vi "Export - Tx Packets.vi"(8 "error in (no error)":errorcluster, 11 "Device Item Ref in":T5 format="%.0x") -> (0 "error out":errorcluster, 3 "Tx Packets":T1 {"Tx Packet Data"."Endianness" items=["big-endian"=0, "little-endian"=2]})   [LabVIEW 2016, in "UDP-Custom-Device System Explorer.lvlib"]
uses:
  UDP-Custom-Device System Explorer.lvlib
  <vilib>/NI Veristand/Custom Device API/Custom Device Item Ref.ctl
  Types/XML - New/ImpExp - Tx Packets Data.ctl
  <vilib>/NI Veristand/Custom Device API/Custom Device Item Info.ctl
  Types/XML - New/ImpExp - Tx Packet Data.ctl
  Shared/Types/Shared - Channel Data Type.ctl
  <vilib>/NI VeriStand/Custom Device API/Custom Device API.lvlib
  Property Accessors/Shared Section Accessors.lvlib
  Shared/UDP-Custom-Device Shared.lvlib
  <vilib>/NI VeriStand/Custom Device Tools/Custom Device Utility Library/Custom Device Utility Library.lvlib
  Property Accessors/Shared Packet Accessors.lvlib
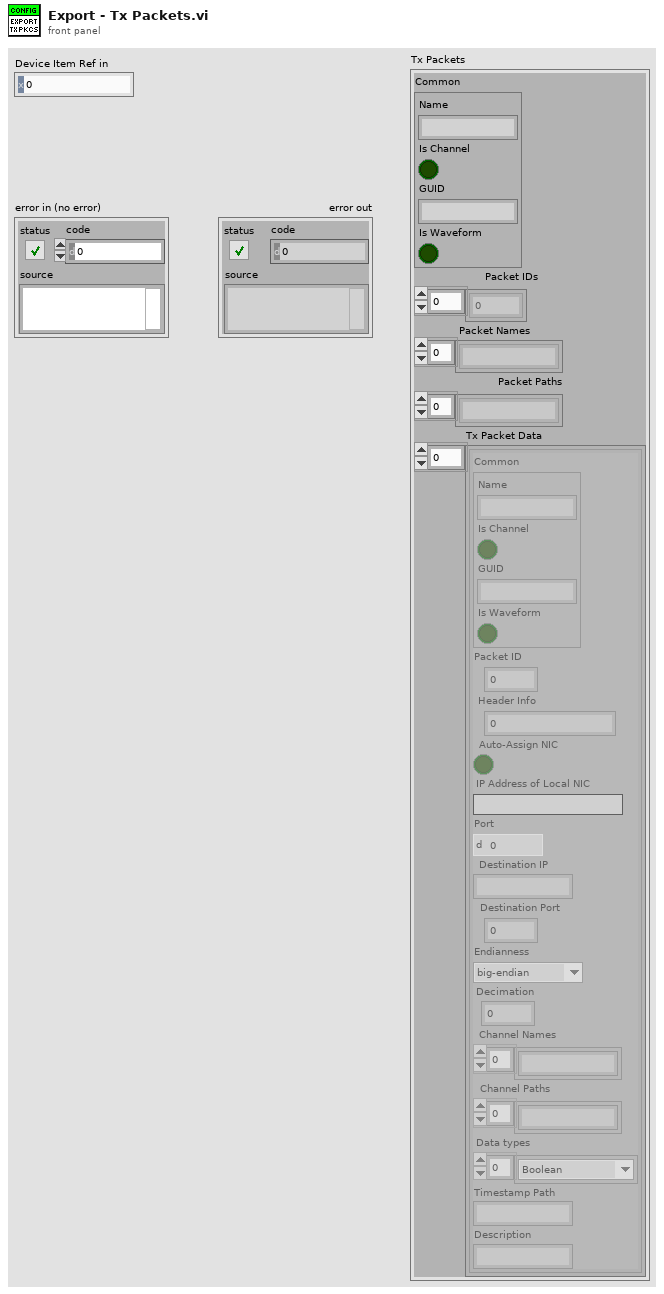
[diagram p1: front panel]
types:
  T1 = typedef "UDP-Custom-Device System Explorer.lvlib/ImpExp - Tx Packets Data.ctl" = cluster{"Common":T2, "Packet IDs":i32[], "Packet Names":string[], "Packet Paths":string[], "Tx Packet Data":T3[]}
  T2 = typedef "Custom Device API.lvlib/Custom Device Item Info.ctl" = cluster{"Name":string, "Is Channel":bool, "GUID":string, "Is Waveform":bool}
  T3 = typedef "UDP-Custom-Device System Explorer.lvlib/ImpExp - Tx Packet Data.ctl" = cluster{"Common":T2, "Packet ID":i32, "Header Info":u32, "Auto-Assign NIC":bool, "IP Address of Local NIC":string, "Port":u16, "Destination IP":string, "Destination Port":u16, "Endianness":u16, "Decimation":u16, "Channel Names":string[], "Channel Paths":string[], "Data types":T4[], "Timestamp Path":string, "Description":string}
  T4 = typedef "UDP-Custom-Device Shared.lvlib/Shared - Channel Data Type.ctl" = enum16{"Boolean", "Single", "Double", "I8", "I16", "I32", "I64", "U8", "U16", "U32", "U64"}
  T5 = typedef "Custom Device API.lvlib/Custom Device Item Ref.ctl" = u64
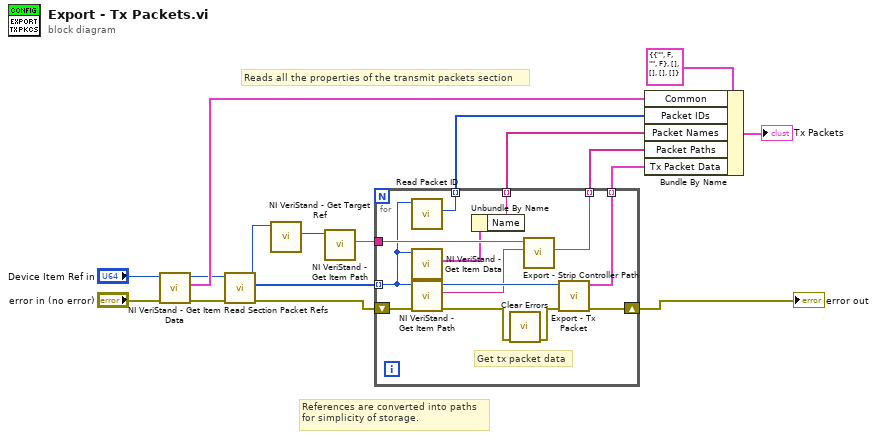
[diagram p0: block diagram]
diagram:
  # "References are converted into paths\nfor simplicity of storage."
  # "Reads all the properties of the transmit packets section"
  n1 = call <vilib>:"NI VeriStand - Get Item Data.vi"("error in (no error)"="error in (no error)", "Item Ref in"="Device Item Ref in") -> ("error out"=w2:errorcluster, "Item Info"=w14:T2, "Item Ref out"=w3:T5)  [unwired: 6 in, 1 out]
  n2 = call "Read Section Packet Refs.vi"("error in (no error)"=w2, "Node Ptr"=w3) -> ("error out"=w12:errorcluster, "Dependent Node Refs"=w10:T5[], "Node Ptr out"=w7:T5)  [unwired: 7 in]
  n3 = call <vilib>:"NI VeriStand - Get Target Ref.vi"("Item Ref in"=w7) -> ("Target Ref"=w8:T5)  [unwired: 7 in, 3 out]
  n4 = call <vilib>:"NI VeriStand - Get Item Path.vi"("Item Ref in"=w8) -> ("Path"=w6:string)  [unwired: 7 in, 3 out]
  n5 = for {
    shift-right: [w28] -> w11
    shift-left: w12 -> [w30]
    tunnel: w10 -> [w21] mode=indexing
    tunnel: [w27] -> w9 mode=indexing
    tunnel: w6 -> [w24]
    tunnel: [w22] -> w5 mode=indexing
    tunnel: [w20] -> w4 mode=indexing
    tunnel: [w18] -> w1 mode=indexing
    # "Get tx packet data"
    n6 = call "Read Packet ID.vi"("Node Ptr"=w21) -> ("Packet ID"=w20:i32)  [unwired: 8 in, 2 out]
    n7 = call <vilib>:"NI VeriStand - Get Item Data.vi"("Item Ref in"=w21) -> ("Item Info"=w19:T2)  [unwired: 7 in, 3 out]
    n8 = call <vilib>:"NI VeriStand - Get Item Path.vi"("error in (no error)"=w30, "Item Ref in"=w21) -> ("error out"=w26:errorcluster, "Path"=w23:string, "Item Ref out"=w29:T5)  [unwired: 6 in, 1 out]
    n9 = Unbundle By Name(w19) -> ("Name"=w18:string)
    n10 = call <vilib>:"Clear Errors.vi"("error in (no error)"=w26) -> ("error out"=w25:errorcluster)  [unwired: 5 in, 1 out]
    n11 = call "Export - Strip Controller Path.vi"("Channel Path"=w23, "Controller Path"=w24) -> ("Stripped Path"=w22:string)  [unwired: 8 in, 1 out]
    n12 = call "Export - Tx Packet.vi"("error in (no error)"=w25, "Device Item Ref in"=w29) -> ("error out"=w28:errorcluster, "Tx Packet"=w27:T3)  [unwired: 8 in]
  }
  "error out" <- w11
  n13 = Bundle By Name(cluster=T1 {"Common"={"Name"="", "Is Channel"=FALSE, "GUID"="", "Is Waveform"=FALSE}, "Packet IDs"=[], "Packet Names"=[], "Packet Paths"=[], "Tx Packet Data"=[]} ("Tx Packets"), "Common"=w14, "Packet IDs"=w4, "Packet Names"=w1, "Packet Paths"=w5, "Tx Packet Data"=w9) -> (→"Tx Packets":T1)
